vi "PCO_Birger.vi"() -> (0 "PCO_Birger":T1, 1 "PCO_Birger_Raw":T2, 2 "Length":u16, 3 "Raw_Length":u16)   [LabVIEW 2019, in "SDK.lvlib" / "Structures.lvlib"]
doc: "Use this template to build a VI to use as a subVI."
uses:
  Structures.lvlib
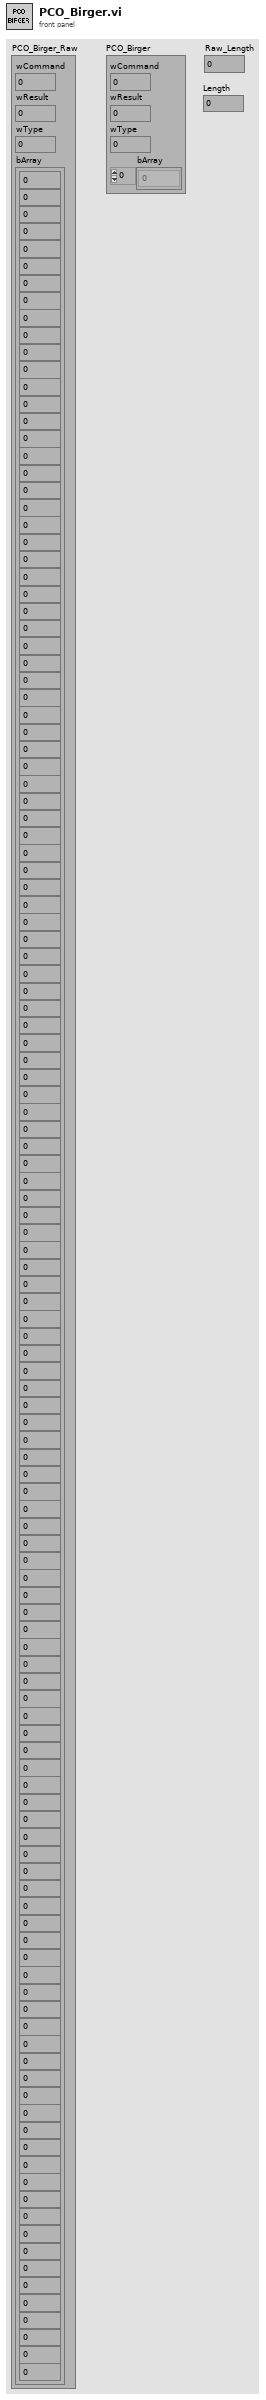
[diagram p1: front panel]
types:
  T1 = cluster{"wCommand":u16, "wResult":u16, "wType":u16, "bArray":u8[]}
  T2 = cluster{"wCommand":u16, "wResult":u16, "wType":u16, "bArray":cluster{u8, u8, u8, u8, u8, u8, u8, u8, u8, u8, u8, u8, u8, u8, u8, u8, u8, u8, u8, u8, u8, u8, u8, u8, u8, u8, u8, u8, u8, u8, u8, u8, u8, u8, u8, u8, u8, u8, u8, u8, u8, u8, u8, u8, u8, u8, u8, u8, u8, u8, u8, u8, u8, u8, u8, u8, u8, u8, u8, u8, u8, u8, u8, u8, u8, u8, u8, u8, u8, u8, u8, u8, u8, u8, u8, u8, u8, u8, u8, u8, u8, u8, u8, u8, u8, u8, u8, u8, u8, u8, u8, u8, u8, u8, u8, u8, u8, u8, u8, u8, u8, u8, u8, u8, u8, u8, u8, u8, u8, u8, u8, u8, u8, u8, u8, u8, u8, u8, u8, u8, u8, u8, u8, u8, u8, u8, u8, u8}}
  T3 = cluster{u8, u8, u8, u8, u8, u8, u8, u8, u8, u8, u8, u8, u8, u8, u8, u8, u8, u8, u8, u8, u8, u8, u8, u8, u8, u8, u8, u8, u8, u8, u8, u8, u8, u8, u8, u8, u8, u8, u8, u8, u8, u8, u8, u8, u8, u8, u8, u8, u8, u8, u8, u8, u8, u8, u8, u8, u8, u8, u8, u8, u8, u8, u8, u8, u8, u8, u8, u8, u8, u8, u8, u8, u8, u8, u8, u8, u8, u8, u8, u8, u8, u8, u8, u8, u8, u8, u8, u8, u8, u8, u8, u8, u8, u8, u8, u8, u8, u8, u8, u8, u8, u8, u8, u8, u8, u8, u8, u8, u8, u8, u8, u8, u8, u8, u8, u8, u8, u8, u8, u8, u8, u8, u8, u8, u8, u8, u8, u8}
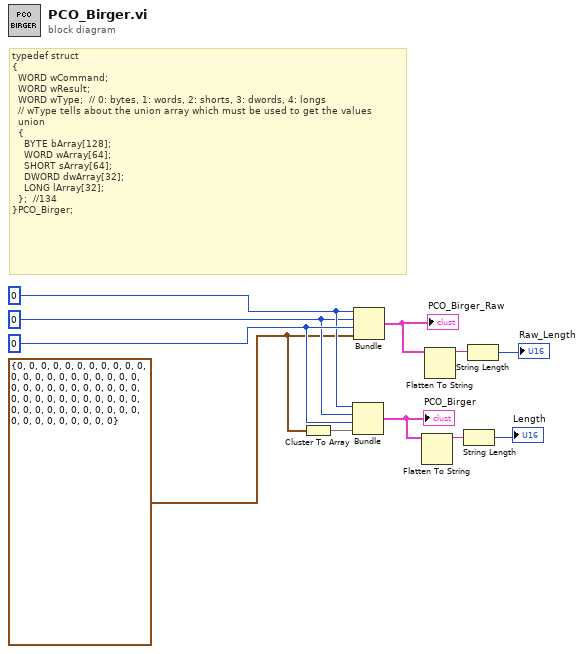
[diagram p0: block diagram]
diagram:
  w1 = T3 {0, 0, 0, 0, 0, 0, 0, 0, 0, 0, 0, 0, 0, 0, 0, 0, 0, 0, 0, 0, 0, 0, 0, 0, 0, 0, 0, 0, 0, 0, 0, 0, 0, 0, 0, 0, 0, 0, 0, 0, 0, 0, 0, 0, 0, 0, 0, 0, 0, 0, 0, 0, 0, 0, 0, 0, 0, 0, 0, 0, 0, 0, 0, 0, 0, 0, 0, 0, 0, 0, 0, 0, 0, 0, 0, 0, 0, 0, 0, 0, 0, 0, 0, 0, 0, 0, 0, 0, 0, 0, 0, 0, 0, 0, 0, 0, 0, 0, 0, 0, 0, 0, 0, 0, 0, 0, 0, 0, 0, 0, 0, 0, 0, 0, 0, 0, 0, 0, 0, 0, 0, 0, 0, 0, 0, 0, 0, 0} ("bArray")
  w6 = u16 0 ("wType")
  w3 = u16 0 ("wResult")
  w4 = u16 0 ("wCommand")
  # "typedef struct  \n{\n  WORD wCommand;\n  WORD wResult;\n  WORD wType;  // 0: bytes, 1: words, 2: shorts, 3: dwords, 4: longs\n  // wType tells about the union array which must be used to get the values\n  union \n  {\n    BYTE bArray[128];\n    WORD wArray[64];\n    SHORT sArray[64];\n    DWORD dwArray[32];\n    LONG lArray[32];\n  };  //134\n}PCO_Birger;"
  n1 = Cluster To Array(cluster=w1) -> (array=w2:u8[])
  n2 = Bundle("wCommand"=w4, "wResult"=w3, "wType"=w6, "bArray"=w2) -> (w5:T1)  [unwired: 1 in]
  "PCO_Birger" <- w5
  n3 = Bundle("wCommand"=w4, "wResult"=w3, "wType"=w6, "bArray"=w1) -> (w7:T2)  [unwired: 1 in]
  "PCO_Birger_Raw" <- w7
  n4 = Flatten To String(anything=w5) -> (data string=w11:string)  [unwired: 3 in, 2 out]
  n5 = Flatten To String(anything=w7) -> (data string=w10:string)  [unwired: 3 in, 2 out]
  n6 = String Length(string=w11) -> (length=→"Length":i32)
  n7 = String Length(string=w10) -> (length=→"Raw_Length":i32)
